vi "Get Uim MCFG wrapper.vi"(8 "error in (no error)":errorcluster caption="错误输入（无错误）", 10 "dwCanNodeId":u32, 11 "dwDevIndex":u32) -> (0 "error out":errorcluster caption="错误输出", 1 "UIM_MCFG_INFO_OBJ":T1, 3 "function return":u32)   [LabVIEW 2016, in "UISimCanFunc_wrapper.lvlib"]
doc: "_declspec (dllexport) DWORD GetUimMCFG_wrapper(DWORD dwDevIndex, DWORD dwCanNodeId, P_DUMMY_UIM_MCFG_INFO_OBJ pDummyMCFGInfo);"
uses:
  <userlib>/UISimCanFunc_wrapper/UISimCanFunc_wrapper.lvlib
  <userlib>/UISimCanFunc_wrapper/ctl/UIM_MCFG_INFO_OBJ.ctl
  <userlib>/UISimCanFunc_wrapper/UISimCanFunc_wrapper.dll
panel:
  in  "pDummyMCFGInfo":T2
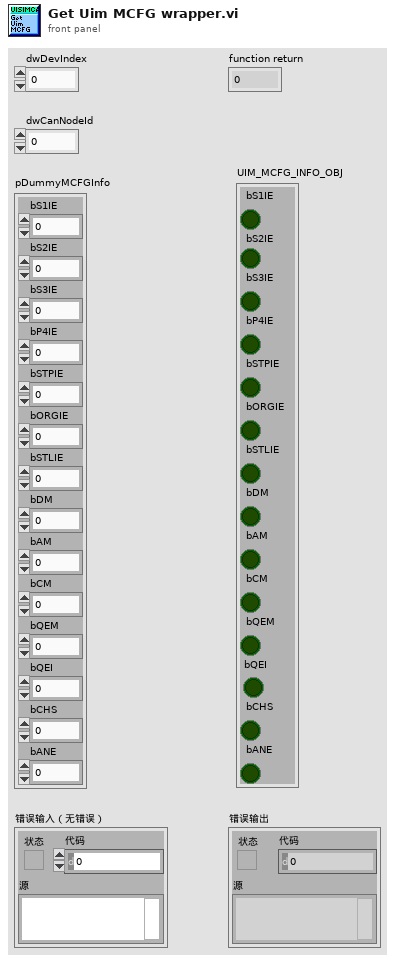
[diagram p1: front panel]
types:
  T1 = typedef "UISimCanFunc_wrapper.lvlib/UIM_MCFG_INFO_OBJ.ctl" = cluster{" bS1IE":bool, " bS2IE":bool, " bS3IE":bool, " bP4IE":bool, " bSTPIE":bool, " bORGIE":bool, " bSTLIE":bool, " bDM":bool, " bAM":bool, " bCM":bool, " bQEM":bool, " bQEI        ":bool, " bCHS":bool, " bANE":bool}
  T2 = cluster{"bS1IE":i32, "bS2IE":i32, "bS3IE":i32, "bP4IE":i32, "bSTPIE":i32, "bORGIE":i32, "bSTLIE":i32, "bDM":i32, "bAM":i32, "bCM":i32, "bQEM":i32, "bQEI":i32, "bCHS":i32, "bANE":i32}
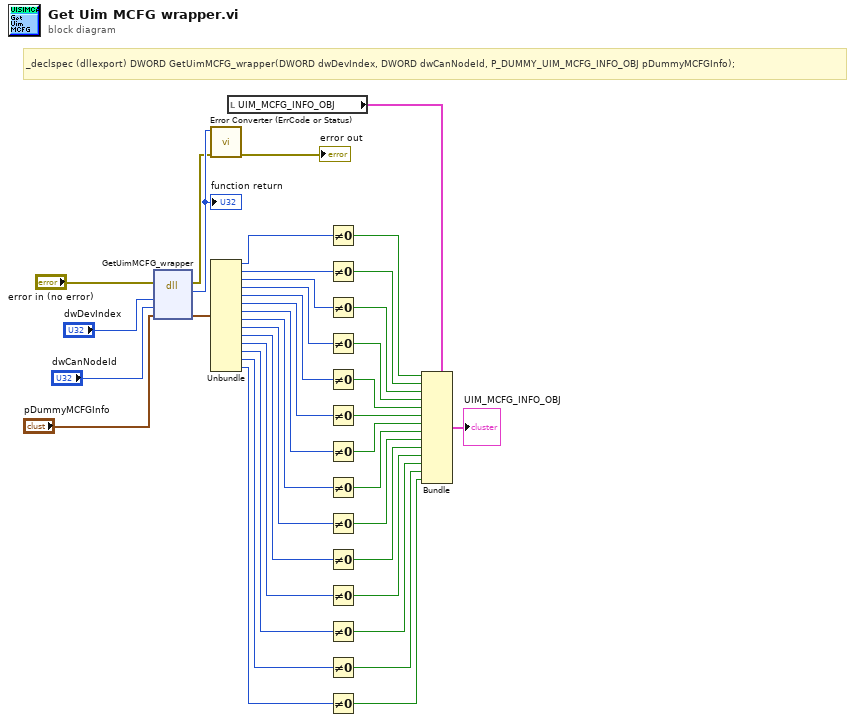
[diagram p0: block diagram]
diagram:
  # "_declspec (dllexport) DWORD GetUimMCFG_wrapper(DWORD dwDevIndex, DWORD dwCanNodeId, P_DUMMY_UIM_MCFG_INFO_OBJ pDummyMCFGInfo);"
  n1 = dll-call lib="C:/Program Files (x86)/National Instruments/LabVIEW 2016/user.lib/UISimCanFunc_wrapper/UISimCanFunc_wrapper.*" fn="GetUimMCFG_wrapper"(error in="error in (no error)", "dwDevIndex"="dwDevIndex", "dwCanNodeId"="dwCanNodeId", "pDummyMCFGInfo"="pDummyMCFGInfo") -> (error out=w33:errorcluster, w38:u32, "pDummyMCFGInfo"=w3:T2)  [unwired: 4 in, 1 out]
  "function return" <- w38
  n2 = call <userlib>:"Error Converter (ErrCode or Status).vi"("error in (no error)"=w33, "error code"=w38) -> ("error out"=→"error out":errorcluster)  [unwired: 9 in]
  n3 = Unbundle(w3) -> ("bS1IE"=w31:i32, "bS2IE"=w29:i32, "bS3IE"=w27:i32, "bP4IE"=w25:i32, "bSTPIE"=w23:i32, "bORGIE"=w21:i32, "bSTLIE"=w19:i32, "bDM"=w17:i32, "bAM"=w15:i32, "bCM"=w13:i32, "bQEM"=w11:i32, "bQEI"=w9:i32, "bCHS"=w7:i32, "bANE"=w5:i32)
  n4 = local read "UIM_MCFG_INFO_OBJ"() -> (w2:T1)
  n5 = Not Equal To 0?(x=w31) -> (x != 0?=w30:bool)
  n6 = Not Equal To 0?(x=w29) -> (x != 0?=w28:bool)
  n7 = Not Equal To 0?(x=w27) -> (x != 0?=w26:bool)
  n8 = Not Equal To 0?(x=w25) -> (x != 0?=w24:bool)
  n9 = Not Equal To 0?(x=w23) -> (x != 0?=w22:bool)
  n10 = Not Equal To 0?(x=w21) -> (x != 0?=w20:bool)
  n11 = Not Equal To 0?(x=w19) -> (x != 0?=w18:bool)
  n12 = Not Equal To 0?(x=w17) -> (x != 0?=w16:bool)
  n13 = Not Equal To 0?(x=w15) -> (x != 0?=w14:bool)
  n14 = Not Equal To 0?(x=w13) -> (x != 0?=w12:bool)
  n15 = Not Equal To 0?(x=w11) -> (x != 0?=w10:bool)
  n16 = Not Equal To 0?(x=w9) -> (x != 0?=w8:bool)
  n17 = Not Equal To 0?(x=w7) -> (x != 0?=w6:bool)
  n18 = Not Equal To 0?(x=w5) -> (x != 0?=w4:bool)
  n19 = Bundle(cluster=w2, "bS1IE"=w30, "bS2IE"=w28, "bS3IE"=w26, "bP4IE"=w24, "bSTPIE"=w22, "bORGIE"=w20, "bSTLIE"=w18, "bDM"=w16, "bAM"=w14, "bCM"=w12, "bQEM"=w10, "bQEI"=w8, "bCHS"=w6, "bANE"=w4) -> (→"UIM_MCFG_INFO_OBJ":T1)
